vi "Finish.vi"(8 "error in (no error)":errorcluster, 11 "System in":refnum<class "System.lvclass">) -> (0 "error out":errorcluster, 3 "System out":refnum<class "System.lvclass">)   [LabVIEW 2013, in "System.lvclass"]
uses:
  System.lvclass
  System.lvclass/System.ctl
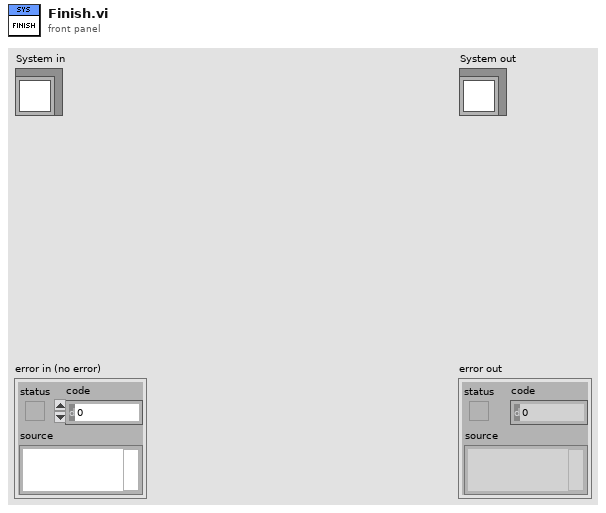
[diagram p1: front panel]
types:
  T1 = typedef "Semaphore RefNum" = refnum<k1>
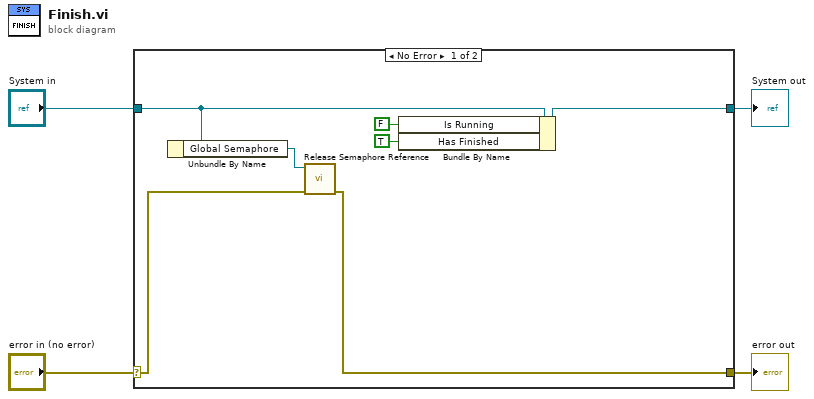
[diagram p0: block diagram]
diagram:
  n1 = case shown="No Error" "error in (no error)" {
    selector: "error in (no error)" -> [w6 w13]
    tunnel: [w5 w13] -> w3
    tunnel: [w11 w12] -> w1
    tunnel: "System in" -> [w8 w12]
    frame No Error {
      n2 = Unbundle By Name(w8) -> ("Global Semaphore"=w7:T1)
      n3 = call <vilib>:"Release Semaphore Reference.vi"("error in (no error)"=w6, "semaphore"=w7) -> ("error out"=w5:errorcluster)  [unwired: 8 in, 1 out]
      n4 = Bundle By Name(cluster=w8, "Is Running"=FALSE ("SystemState.Is Running"), "Has Finished"=TRUE ("SystemState.Has Finished")) -> (w11:refnum<class "System.lvclass">)
    }
    frame Error {
    }
  }
  "error out" <- w3
  "System out" <- w1
